vi "Read Charact Standard List.vi"(8 "error in (no error)":errorcluster, 11 "SA 18GHz Path Group in":refnum<class "SA 18GHz Path Group.lvclass">) -> (0 "error out":errorcluster, 2 "Charact Standard List":T1[](array[typedef]), 3 "SA 18GHz Path Group out":refnum<class "SA 18GHz Path Group.lvclass">)   [LabVIEW 2023, in "RFFixtureCharact.RFPM.lvlib" / "SA 18GHz Path Group.lvclass"]
uses:
  SA 18GHz Path Group.lvclass
  Instruments/Cal Standard/Type Definitions/Standard Type.ctl
  Instruments/RFFixtureCharact.Instruments.lvlib
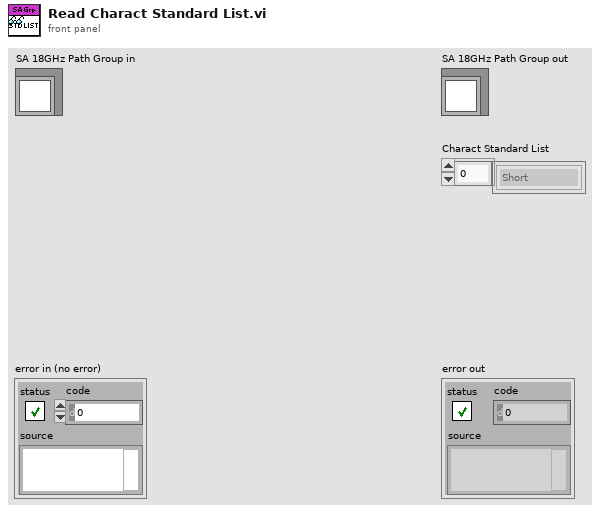
[diagram p1: front panel]
types:
  T1 = typedef "RFFixtureCharact.Instruments.lvlib/Standard Type.ctl" = enum16{"Short", "Open", "Load", "PowerMeter", "None"}
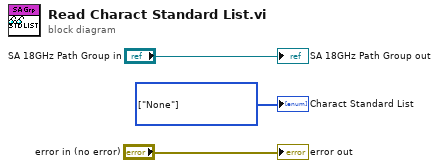
[diagram p0: block diagram]
diagram:
  w1 = T1[] [enum."None"] items=["Short", "Open", "Load", "PowerMeter", "None"] ("Charact Standard List")
  "error out" <- "error in (no error)"
  "SA 18GHz Path Group out" <- "SA 18GHz Path Group in"
  "Charact Standard List" <- w1
